vi "Main_Loop.vi"(6 "Queues":T1, 7 "Timer parameters":refnum<vi>, 8 "Status/Errors in":refnum<vi>, 9 "Control Parameters [] in":T2[](array[typedef]) {"Aux Byte Value" format="%02x"; "Max Real Value" format="%#_6e"; "Min Real Value" format="%#_6e"; "dReal/dByte" format="%#_6e"; "Byte Value" format="%02x"; "Identifier" format="%02x"}, 10 "Main parameters in":T5={"Mode"={"Mode"=enum."Dialog", "Expert?"=FALSE, "Dialog?"=FALSE}, "Stop loop"={"Settings changed?"=FALSE, "Stop?"=refnum}, "Send message"={"Send mode"=enum."Get parameters", "Set parameter list"=0, "Get parameter list"=0, "Reset device"=0, "Length set settings message"=0, "Reset buttons?"=FALSE, "Reset Master?"=enum."General"}, "Write settings"={"Options"=enum."File 1"}, "Settings state"={"MAS locked?"=refnum, "SLV locked?"=refnum}, "Button refs"={"Stop program"=refnum, "Save settings"=refnum, "DAQ mode"=refnum, "Reset settings"=refnum, "Apply settings"=refnum, "Reset MAS"=refnum, "Reset SLV"=refnum, "Local DBase?"=refnum, "Last value DBase"=FALSE, "Database"=refnum, "Calibration"=refnum, "Save settings 2"=refnum}, "Update screen"={"Detector number"=0, "Hardware"=enum."None"}, "Files"={"Path config file"=path "", "Path def. ini file"=path "", "Path ini file 1"=path "", "Path ini file 2"=path "", "Path RBF file"=path ""}, "DB connection"={"connection reference"=refnum, "Connected?"=refnum, "ODBC Name"=""}, "Status_id"=refnum, "Time difference"=refnum, "Satellites"=refnum, "Alignment parameters"=refnum, "Page Statistics 2"=refnum, "Database"=refnum, "Page Statistics"=refnum} {"Update screen"."Detector number" format="%#.0f"; "Send message"."Reset device" format="%x"; "Send message"."Get parameter list" format="%x"; "Send message"."Set parameter list" format="%x"}, 11 "Devices in":T4) -> (0 "Status/Errors out":refnum<vi>, 1 "Control Parameters [] out":T2[](array[typedef]) {"Aux Byte Value" format="%02x"; "Max Real Value" format="%#_6e"; "Min Real Value" format="%#_6e"; "dReal/dByte" format="%#_6e"; "Byte Value" format="%02x"; "Identifier" format="%02x"}, 2 "Main parameters out":T5={"Mode"={"Mode"=enum."Dialog", "Expert?"=FALSE, "Dialog?"=FALSE}, "Stop loop"={"Settings changed?"=FALSE, "Stop?"=refnum}, "Send message"={"Send mode"=enum."Get parameters", "Set parameter list"=0, "Get parameter list"=0, "Reset device"=0, "Length set settings message"=0, "Reset buttons?"=FALSE, "Reset Master?"=enum."General"}, "Write settings"={"Options"=enum."File 1"}, "Settings state"={"MAS locked?"=refnum, "SLV locked?"=refnum}, "Button refs"={"Stop program"=refnum, "Save settings"=refnum, "DAQ mode"=refnum, "Reset settings"=refnum, "Apply settings"=refnum, "Reset MAS"=refnum, "Reset SLV"=refnum, "Local DBase?"=refnum, "Last value DBase"=FALSE, "Database"=refnum, "Calibration"=refnum, "Save settings 2"=refnum}, "Update screen"={"Detector number"=0, "Hardware"=enum."None"}, "Files"={"Path config file"=path "", "Path def. ini file"=path "", "Path ini file 1"=path "", "Path ini file 2"=path "", "Path RBF file"=path ""}, "DB connection"={"connection reference"=refnum, "Connected?"=refnum, "ODBC Name"=""}, "Status_id"=refnum, "Time difference"=refnum, "Satellites"=refnum, "Alignment parameters"=refnum, "Page Statistics 2"=refnum, "Database"=refnum, "Page Statistics"=refnum} {"Update screen"."Detector number" format="%#.0f"; "Send message"."Reset device" format="%x"; "Send message"."Get parameter list" format="%x"; "Send message"."Set parameter list" format="%x"})   [LabVIEW 2013]
uses:
  Controls/Main_Parameters.ctl
  Controls/Mode.ctl
  Controls/Stop_Loop.ctl
  Controls/Send_Message.ctl
  Controls/Send_Message_Mode.ctl
  Controls/Master.ctl
  Controls/Write_Settings.ctl
  Controls/Write_Settings_Options.ctl
  Controls/Settings_State.ctl
  Controls/Button_Refs.ctl
  Controls/Update_Screen.ctl
  Controls/Files.ctl
  Controls/DB_Connection.ctl
  database/Connection.llb/Conn ObjectReference.ctl
  Controls/Devices.ctl
  Controls/Control_Parameters.ctl
  Controls/Queues.ctl
  Controls/One_Second.ctl
  Controls/GPS_Timestamp.ctl
  Controls/Get_Set_Buttons_mode.ctl
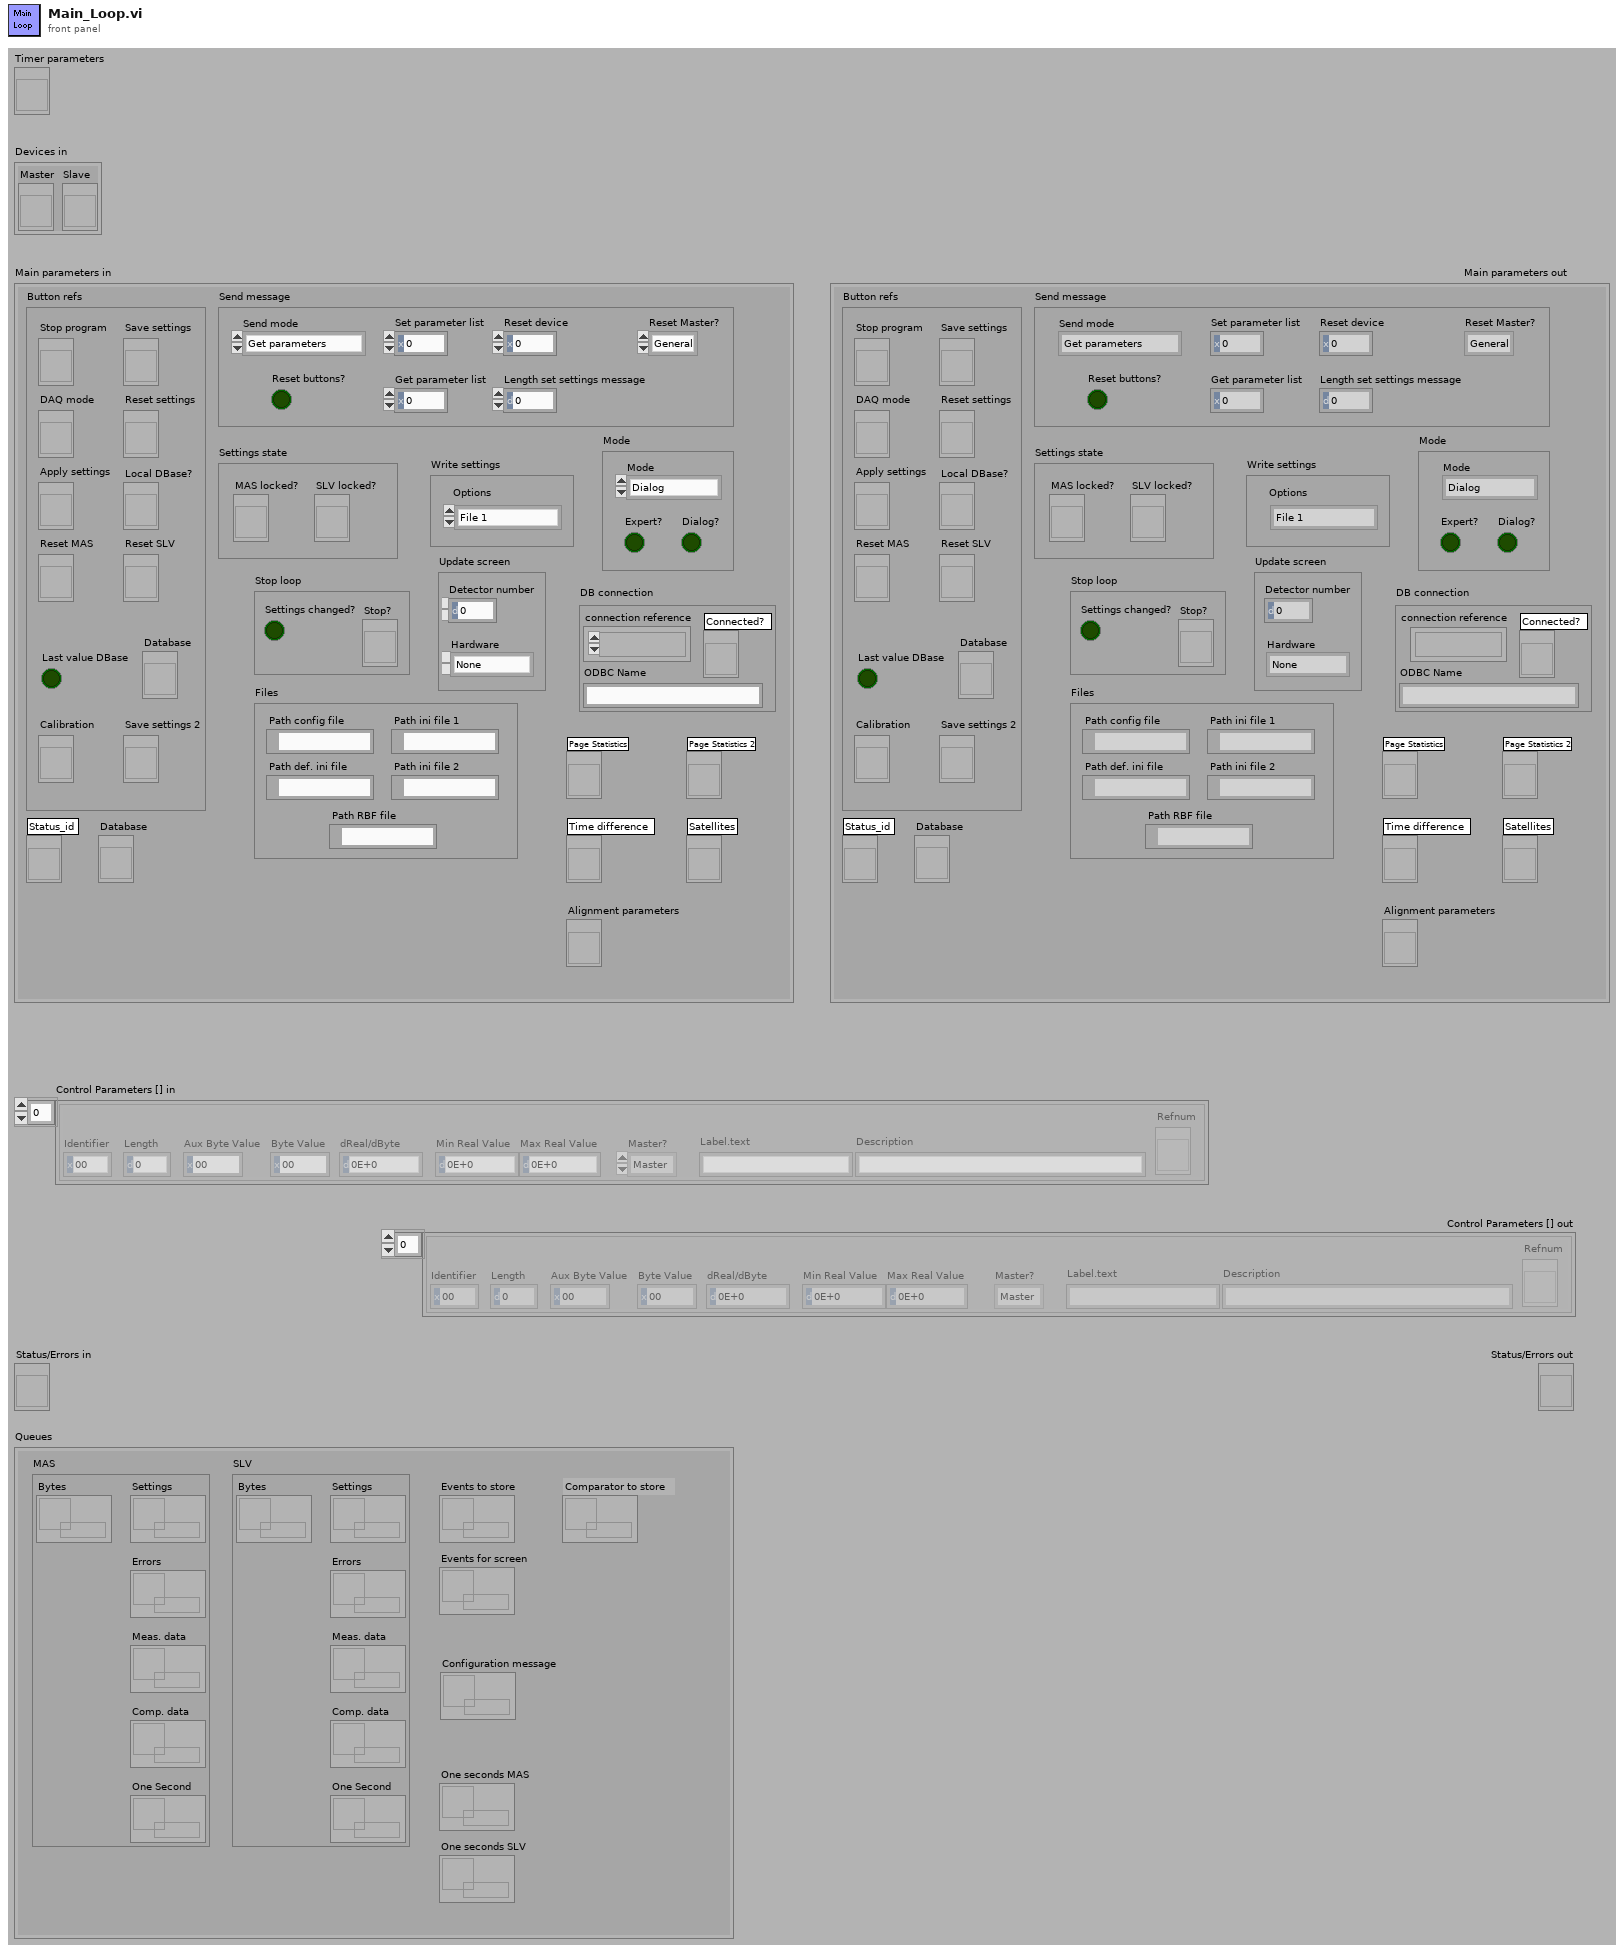
[diagram p1: front panel]
types:
  T1 = typedef "Queues.ctl" = cluster{"MAS":cluster{"Bytes":refnum<queue>, "Settings":refnum<queue>, "Errors":refnum<queue>, "Meas. data":refnum<queue>, "One Second":refnum<queue>, "Comp. data":refnum<queue>}, "SLV":cluster{"Bytes":refnum<queue>, "Settings":refnum<queue>, "Errors":refnum<queue>, "Meas. data":refnum<queue>, "One Second":refnum<queue>, "Comp. data":refnum<queue>}, "Events to store":refnum<queue>, "Events for screen":refnum<queue>, "One seconds MAS":refnum<queue>, "One seconds SLV":refnum<queue>, "Configuration message":refnum<queue>, "Comparator to store":refnum<queue>}
  T2 = typedef "Control_Parameters.ctl" = cluster{"Identifier":u8, "Length":u16, "Byte Value":u32, "dReal/dByte":dbl, "Min Real Value":dbl, "Max Real Value":dbl, "Master?":T3, "Label.text":string, "Description":string, "Refnum":refnum<vi>, "Aux Byte Value":u32}
  T3 = typedef "Master.ctl" = enum16{"Master", "Slave", "General"}
  T4 = typedef "Devices.ctl" = cluster{"Master":refnum<vi>, "Slave":refnum<vi>}
  T5 = typedef "Main_Parameters.ctl" = cluster{"Mode":T6, "Stop loop":T7, "Send message":T8, "Write settings":T10, "Settings state":T12, "Button refs":T13, "Update screen":T14, "Files":T15, "DB connection":T16, "Status_id":refnum<vi>, "Time difference":refnum<vi>, "Satellites":refnum<vi>, "Alignment parameters":refnum<vi>, "Page Statistics 2":refnum<vi>, "Database":refnum<vi>, "Page Statistics":refnum<vi>}
  T6 = typedef "Mode.ctl" = cluster{"Mode":enum8{"Stop", "Dialog", "Hisparc II", "Hisparc II DAQ", "Alignment"}, "Expert?":bool, "Dialog?":bool}
  T7 = typedef "Stop_Loop.ctl" = cluster{"Settings changed?":bool, "Stop?":refnum<vi>}
  T8 = typedef "Send_Message.ctl" = cluster{"Send mode":T9, "Set parameter list":u8, "Get parameter list":u8, "Reset device":u8, "Length set settings message":i32, "Reset buttons?":bool, "Reset Master?":T3}
  T9 = typedef "Send_Message_Mode.ctl" = enum16{"Get parameters", "Set parameters", "From front panel", "From parameters", "Reset device", "Alignment"}
  T10 = typedef "Write_Settings.ctl" = cluster{"Options":T11}
  T11 = typedef "Write_Settings_Options.ctl" = enum16{"File 1", "File 2", "Alignment", "Reset"}
  T12 = typedef "Settings_State.ctl" = cluster{"MAS locked?":refnum<vi>, "SLV locked?":refnum<vi>}
  T13 = typedef "Button_Refs.ctl" = cluster{"Stop program":refnum<vi>, "Save settings":refnum<vi>, "DAQ mode":refnum<vi>, "Reset settings":refnum<vi>, "Apply settings":refnum<vi>, "Reset MAS":refnum<vi>, "Reset SLV":refnum<vi>, "Local DBase?":refnum<vi>, "Last value DBase":bool, "Database":refnum<vi>, "Calibration":refnum<vi>, "Save settings 2":refnum<vi>}
  T14 = typedef "Update_Screen.ctl" = cluster{"Detector number":u16, "Hardware":enum8{"None", "HiSPARC I", "HiSPARC II", "HiSPARC III", "Unknown"}}
  T15 = typedef "Files.ctl" = cluster{"Path config file":path, "Path def. ini file":path, "Path ini file 1":path, "Path ini file 2":path, "Path RBF file":path}
  T16 = typedef "DB_Connection.ctl" = cluster{"connection reference":T17, "Connected?":refnum<vi>, "ODBC Name":string}
  T17 = typedef "Conn ObjectReference.ctl" = refnum<k1>
  T18 = typedef "Get_Set_Buttons_mode.ctl" = enum16{"Get", "Get DAQ", "Set", "Set settings"}
  T19 = typedef "Command_Main_Loop.ctl" = enum16{"Send message", "Check settings", "Update screen", "Write settings", "Stop loop", "No action"}
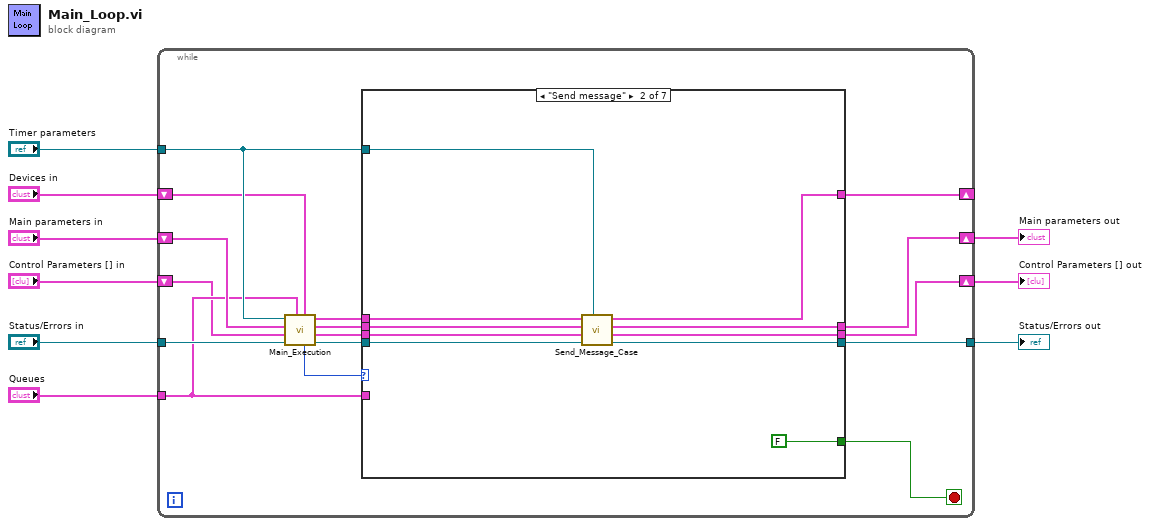
[diagram p0: block diagram]
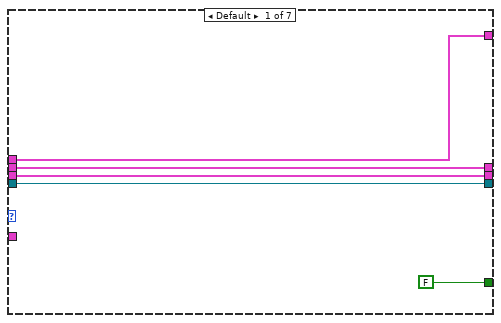
[diagram p2: hidden frame]
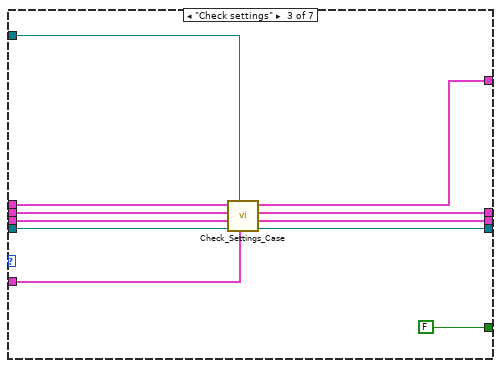
[diagram p3: hidden frame]
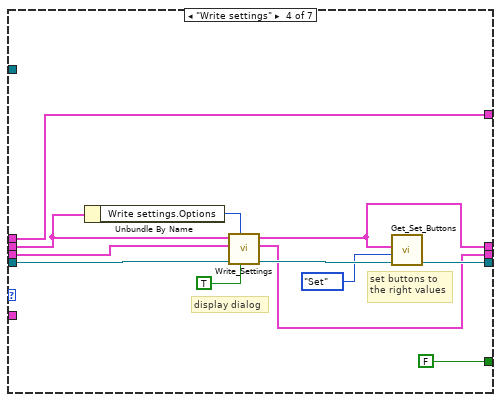
[diagram p4: hidden frame]
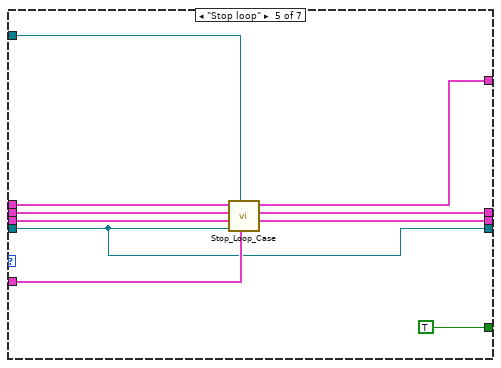
[diagram p5: hidden frame]
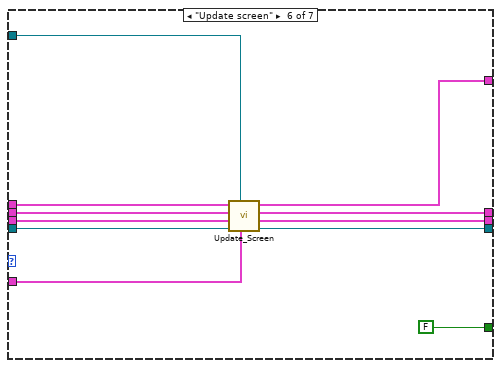
[diagram p6: hidden frame]
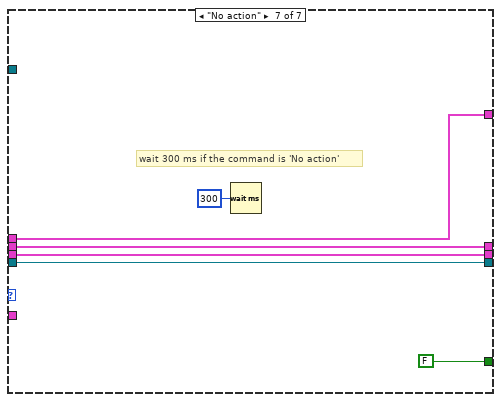
[diagram p7: hidden frame]
diagram:
  n1 = while {
    tunnel: "Status/Errors in" -> [w23]
    tunnel: [w20] -> w6
    tunnel: "Timer parameters" -> [w19]
    shift-right: [w16] -> w4
    shift-left: "Main parameters in" -> [w22]
    shift-right: [w15] -> _
    shift-left: "Devices in" -> [w18]
    shift-right: [w14] -> w3
    shift-left: "Control Parameters [] in" -> [w12]
    tunnel: "Queues" -> [w13]
    stop <- w17 stop-if-true
    n2 = call "Main_Execution.vi"("Devices in"=w18, "Queues"=w13, "Status/Errors in"=w23, "Control Parameters [] in"=w12, "Main parameters in"=w22, "Timer parameters"=w19) -> ("Status/Errors out"=w24:refnum<vi>, "Control Parameters [] out"=w25:T2[], "Main parameters out"=w10:T5, "Devices out"=w11:T4, "Command"=w21:T19)  [unwired: 1 in]
    n3 = case shown="\"Send message\"" w21 {
      tunnel: w24 -> [w30 w39 w50 w63 w65 w81 w88]
      tunnel: [w30 w38 w49 w58 w65 w79 w88] -> w20
      tunnel: w25 -> [w29 w36 w44 w61 w73 w84 w87]
      tunnel: [w29 w37 w43 w54 w68 w82 w87] -> w14
      tunnel: w10 -> [w28 w35 w45 w62 w72 w78 w86]
      tunnel: [w28 w34 w42 w55 w67 w77 w86] -> w16
      tunnel: w11 -> [w26 w31 w46 w57 w71 w76 w85]
      tunnel: [w26 w32 w41 w57 w66 w75 w85] -> w15
      tunnel: [FALSE FALSE ("Stop Loop?") FALSE ("Stop Loop?") FALSE ("Stop Loop?") TRUE ("Stop Loop?") FALSE ("Stop Loop?") FALSE ("Stop Loop?")] -> w17
      tunnel: w19 -> [_ w33 w47 _ w70 w74 _]
      tunnel: w13 -> [_ _ w48 _ w69 w83 _]
      frame Default {
      }
      frame "Send message" {
        n4 = call "Send_Message_Case.vi"("Timer parameters"=w33, "Status/Errors in"=w39, "Control Parameters [] in"=w36, "Main parameters in"=w35, "Devices in"=w31) -> ("Status/Errors out"=w38:refnum<vi>, "Control Parameters [] out"=w37:T2[], "Main parameters out"=w34:T5, "Devices out"=w32:T4)  [unwired: 1 in, 2 out]
      }
      frame "Check settings" {
        n5 = call "Check_Settings_Case.vi"("Queues"=w48, "Timer parameters"=w47, "Status/Errors in"=w50, "Control Parameters [] in"=w44, "Main parameters in"=w45, "Devices in"=w46) -> ("Status/Errors out"=w49:refnum<vi>, "Control Parameters [] out"=w43:T2[], "Main parameters out"=w42:T5, "Devices out"=w41:T4)  [unwired: 2 out]
      }
      frame "Write settings" {
        # "set buttons to\nthe right values"
        # "display dialog"
        n6 = Unbundle By Name(w62) -> ("Write settings.Options"=w52:T11)
        n7 = call "Write_Settings.vi"("Dialog? (false)"=TRUE, "Options"=w52, "Status/Errors in"=w63, "Control Parameters [] in"=w61, "Main parameters in"=w62) -> ("Status/Errors out"=w56:refnum<vi>, "Control Parameters [] out"=w54:T2[], "Main parameters out"=w55:T5)  [unwired: 4 out]
        n8 = call "Get_Set_Buttons.vi"("Status/Errors in"=w56, "Set?"=Get_Set_Buttons_mode."Set", "Main parameters"=w55) -> ("Status/Errors out"=w58:refnum<vi>)  [unwired: 1 in, 7 out]
      }
      frame "Stop loop" {
        n9 = call "Stop_Loop_Case.vi"("Queues"=w69, "Timer parameters"=w70, "Status/Errors in"=w65, "Control Parameters [] in"=w73, "Main parameters in"=w72, "Devices in"=w71) -> ("Control Parameters [] out"=w68:T2[], "Main parameters out"=w67:T5, "Devices out"=w66:T4)  [unwired: 3 out]
      }
      frame "Update screen" {
        n10 = call "Update_Screen.vi"("Queues"=w83, "Timer parameters"=w74, "Status/Errors in"=w81, "Control Parameters [] in"=w84, "Main parameters in"=w78, "Devices in"=w76) -> ("Status/Errors out"=w79:refnum<vi>, "Control Parameters [] out"=w82:T2[], "Main parameters out"=w77:T5, "Devices out"=w75:T4)  [unwired: 2 in]
      }
      frame "No action" {
        # "wait 300 ms if the command is 'No action'"
        n11 = Wait (ms)(milliseconds to wait=u32 300) -> ()  [unwired: 1 out]
      }
    }
  }
  "Status/Errors out" <- w6
  "Main parameters out" <- w4
  "Control Parameters [] out" <- w3
